vi "DevRef Data Base fg.vi"(6 "DevRef to Get":T11, 9 "Menu":T12) -> (0 "error out":errorcluster, 1 "Selected Sensor":T5, 2 "Selected Encoder":T1={"DevStatus"={"status"=FALSE, "code"=0, "source"=""}, "EncoderIndex"=enum."Invalid", "CounterIndex"=enum."Invalid", "DistancePerCount"=1.0, "Decoding Type"=enum."4x"}, 3 "Selected Solenoid":T8={"DevStatus"={"status"=FALSE, "code"=0, "source"=""}, "Solenoid Module"=enum."Solenoid Module 1", "Forward Solenoid Channel"=enum."Invalid", "Reverse Solenoid Channel"=enum."Invalid"}, 4 "right drive encoder":T1={"DevStatus"={"status"=FALSE, "code"=0, "source"=""}, "EncoderIndex"=enum."Invalid", "CounterIndex"=enum."Invalid", "DistancePerCount"=1.0, "Decoding Type"=enum."4x"}, 5 "left drive encoder":T1={"DevStatus"={"status"=FALSE, "code"=0, "source"=""}, "EncoderIndex"=enum."Invalid", "CounterIndex"=enum."Invalid", "DistancePerCount"=1.0, "Decoding Type"=enum."4x"})   [LabVIEW 2013]
uses:
  typedefs/fg_typedef.ctl
  typedefs/DevRef Type.ctl
  <vilib>/Rock Robotics/WPI/Solenoid/WPI_SolenoidDevRef.ctl
  <vilib>/Rock Robotics/SystemInterfaces/Typedef/FPGA_TypedefSolenoidModule.ctl
  <vilib>/Rock Robotics/WPI/Solenoid/WPI_SolenoidChannel.ctl
  <vilib>/Rock Robotics/WPI/DigitalInput/WPI_DigitalInputDevRef.ctl
  <vilib>/Rock Robotics/SystemInterfaces/DIO/FPGA_DIOChannel.ctl
  <vilib>/Rock Robotics/SystemInterfaces/Typedef/FPGA_TypedefDigitalModule.ctl
  <vilib>/Rock Robotics/WPI/Encoder/WPI_EncoderDevRef.ctl
  <vilib>/Rock Robotics/SystemInterfaces/Encoder/FPGA_EncoderIdx.ctl
  <vilib>/Rock Robotics/SystemInterfaces/Counter/FPGA_CounterCtrSystemIndex.ctl
  <vilib>/Rock Robotics/WPI/Encoder/WPI_EncoderType.ctl
panel:
  # "A Functional Global that stores refnums for \ncommonly used devices \nso as to not need to get them repeatedly"
  # "it is only set once"
  # "Option to Select Also..."
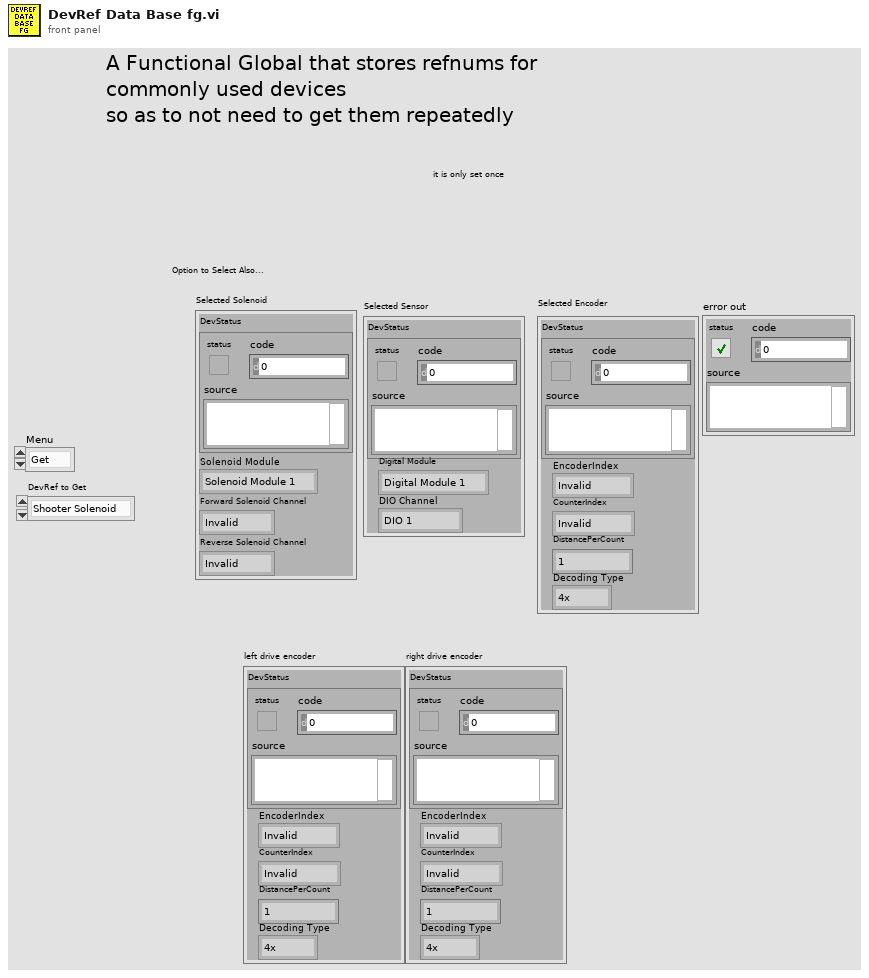
[diagram p1: front panel]
types:
  T1 = typedef "WPI_EncoderDevRef.ctl" = cluster{"DevStatus":errorcluster, "EncoderIndex":T2, "CounterIndex":T3, "DistancePerCount":dbl, "Decoding Type":T4}
  T2 = typedef "FPGA_EncoderIdx.ctl" = enum8{"Enc 0", "Enc 1", "Enc 2", "Enc 3", "Invalid"}
  T3 = typedef "FPGA_CounterCtrSystemIndex.ctl" = enum8{"Ctr 0", "Ctr 1", "Ctr 2", "Ctr 3", "Ctr 4", "Ctr 5", "Ctr 6", "Ctr 7", "Invalid"}
  T4 = typedef "WPI_EncoderType.ctl" = enum16{"1x", "2x", "4x"}
  T5 = typedef "WPI_DigitalInputDevRef.ctl" = cluster{"DevStatus":errorcluster, "DIO Channel":T6, "Digital Module":T7}
  T6 = typedef "FPGA_DIOChannel.ctl" = enum8{"DIO 1", "DIO 2", "DIO 3", "DIO 4", "DIO 5", "DIO 6", "DIO 7", "DIO 8", "DIO 9", "DIO 10", "DIO 11", "DIO 12", "DIO 13", "DIO 14", "Invalid"}
  T7 = typedef "FPGA_TypedefDigitalModule.ctl" = enum16{"Digital Module 1", "Digital Module 2"}
  T8 = typedef "WPI_SolenoidDevRef.ctl" = cluster{"DevStatus":errorcluster, "Solenoid Module":T9, "Forward Solenoid Channel":T10, "Reverse Solenoid Channel":T10}
  T9 = typedef "FPGA_TypedefSolenoidModule.ctl" = enum16{"Solenoid Module 1", "Solenoid Module 2"}
  T10 = typedef "WPI_SolenoidChannel.ctl" = enum8{"Solenoid 1", "Solenoid 2", "Solenoid 3", "Solenoid 4", "Solenoid 5", "Solenoid 6", "Solenoid 7", "Solenoid 8", "Invalid"}
  T11 = typedef "DevRef Type.ctl" = enum16{"Shooter Solenoid", "Latch Solenoid", "Right Up Sensor", "Right Down Sensor", "Hold Sensor", "2 Ball Switch", "Arm Encoder"}
  T12 = typedef "fg_typedef.ctl" = enum16{"Get", "Set"}
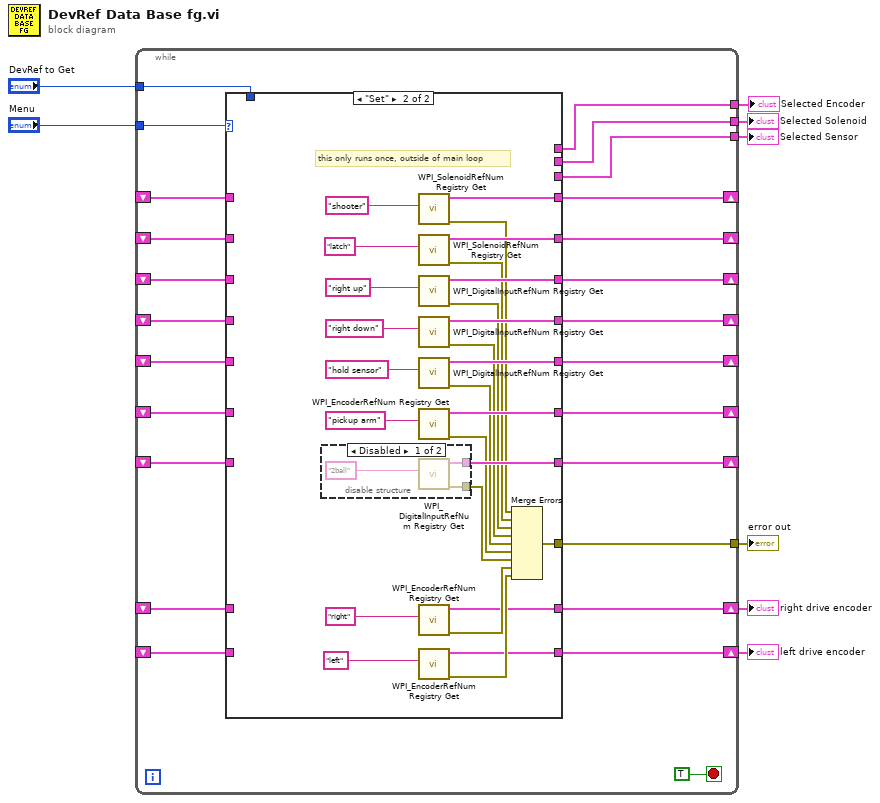
[diagram p0: block diagram]
diagram:
  n1 = while {
    shift-right: [w27] -> _
    shift-left: _ -> [w32]
    shift-right: [w26] -> _
    shift-left: _ -> [w31]
    shift-right: [w25] -> _
    shift-left: _ -> [w29]
    shift-right: [w24] -> _
    shift-left: _ -> [w28]
    tunnel: "Menu" -> [w30]
    shift-right: [w22] -> _
    shift-left: _ -> [w23]
    tunnel: "DevRef to Get" -> [w21]
    tunnel: [w20] -> w6
    tunnel: [w19] -> w5
    shift-right: [w17] -> _
    shift-left: _ -> [w18]
    tunnel: [w16] -> w4
    shift-right: [w15] -> _
    shift-left: _ -> [w14]
    shift-right: [w13] -> w2
    shift-left: _ -> [w10]
    shift-right: [w12] -> w1
    shift-left: _ -> [w9]
    tunnel: [w11] -> w3
    stop <- TRUE stop-if-true
    n2 = case shown="\"Set\"" w30 {
      tunnel: w32 -> [w52 _]
      tunnel: w31 -> [w51 _]
      tunnel: w29 -> [w50 _]
      tunnel: w28 -> [w49 _]
      tunnel: [w41 w124] -> w27
      tunnel: [w42 w123] -> w26
      tunnel: [w43 w122] -> w25
      tunnel: [w44 w121] -> w24
      tunnel: w23 -> [w48 _]
      tunnel: [w45 w120] -> w22
      tunnel: w21 -> [w53 _]
      tunnel: [w47 _] -> w20
      tunnel: [w46 _] -> w19
      tunnel: w18 -> [w40 _]
      tunnel: [w39 w118] -> w17
      tunnel: [w38 _] -> w16
      tunnel: [w37 w117] -> w15
      tunnel: w14 -> [w36 _]
      tunnel: [w35 w105] -> w13
      tunnel: [w34 w104] -> w12
      tunnel: [_ w103] -> w11
      tunnel: w10 -> [w35 _]
      tunnel: w9 -> [w34 _]
      frame "Get", Default {
        # "always get the drive encoders"
        n3 = case shown="\"Shooter Solenoid\", Default" w53 {
          tunnel: w52 -> [w56 w67 w74 w81 w88 w90 w102]
          tunnel: w51 -> [w57 w66 w73 w80 w87 w91 w101]
          tunnel: w50 -> [w58 w65 w72 w79 w86 w92 w100]
          tunnel: w49 -> [w59 w64 w71 w78 w85 w93 w99]
          tunnel: w48 -> [w60 w63 w70 w77 w84 w94 w98]
          tunnel: [w56 w66 _ _ _ _ _] -> w47
          tunnel: [_ _ w72 w78 w84 w89 _] -> w46
          tunnel: [w60 w63 w70 w77 w84 w94 w98] -> w45
          tunnel: [w59 w64 w71 w78 w85 w93 w99] -> w44
          tunnel: [w58 w65 w72 w79 w86 w92 w100] -> w43
          tunnel: [w57 w66 w73 w80 w87 w91 w101] -> w42
          tunnel: [w56 w67 w74 w81 w88 w90 w102] -> w41
          tunnel: w40 -> [w55 w62 w69 w76 w83 w95 w97]
          tunnel: [w55 w62 w69 w76 w83 w95 w97] -> w39
          tunnel: [_ _ _ _ _ _ w97] -> w38
          tunnel: [w54 w61 w68 w75 w82 w89 w96] -> w37
          tunnel: w36 -> [w54 w61 w68 w75 w82 w89 w96]
          frame "Shooter Solenoid", Default {
          }
          frame "Latch Solenoid" {
          }
          frame "Right Up Sensor" {
          }
          frame "Right Down Sensor" {
          }
          frame "Hold Sensor" {
          }
          frame "2 Ball Switch" {
          }
          frame "Arm Encoder" {
          }
        }
      }
      frame "Set" {
        # "this only runs once, outside of main loop"
        n4 = disable-structure shown="Disabled" {
          disable-tunnel: [w132 _] -> w110
          disable-tunnel: [w130 _] -> w117
          frame Disabled {
            n5 = call <vilib>:"WPI_DigitalInputRefNum Registry Get.vi"("refnum name"="2ball") -> ("error out"=w132:errorcluster, "DigitalInputDevRef"=w130:T5)  [unwired: 9 in]
          }
          frame Enabled {
          }
        }
        n6 = call <vilib>:"WPI_SolenoidRefNum Registry Get.vi"("refnum name"="shooter") -> ("error out"=w116:errorcluster, "SolenoidDevRef"=w124:T8)  [unwired: 9 in]
        n7 = call <vilib>:"WPI_SolenoidRefNum Registry Get.vi"("refnum name"="latch") -> ("error out"=w115:errorcluster, "SolenoidDevRef"=w123:T8)  [unwired: 9 in]
        n8 = call <vilib>:"WPI_DigitalInputRefNum Registry Get.vi"("refnum name"="right up") -> ("error out"=w114:errorcluster, "DigitalInputDevRef"=w122:T5)  [unwired: 9 in]
        n9 = call <vilib>:"WPI_DigitalInputRefNum Registry Get.vi"("refnum name"="right down") -> ("error out"=w113:errorcluster, "DigitalInputDevRef"=w121:T5)  [unwired: 9 in]
        n10 = call <vilib>:"WPI_DigitalInputRefNum Registry Get.vi"("refnum name"="hold sensor") -> ("error out"=w112:errorcluster, "DigitalInputDevRef"=w120:T5)  [unwired: 9 in]
        n11 = call <vilib>:"WPI_EncoderRefNum Registry Get.vi"("refnum name"="pickup arm") -> ("error out"=w111:errorcluster, "EncoderDevRef"=w118:T1)  [unwired: 9 in]
        n12 = call <vilib>:"WPI_EncoderRefNum Registry Get.vi"("refnum name"="right") -> ("error out"=w107:errorcluster, "EncoderDevRef"=w105:T1)  [unwired: 9 in]
        n13 = call <vilib>:"WPI_EncoderRefNum Registry Get.vi"("refnum name"="left") -> ("error out"=w106:errorcluster, "EncoderDevRef"=w104:T1)  [unwired: 9 in]
        n14 = Merge Errors(w116, w115, w114, w113, w112, w111, w110, w107, w106) -> (w103:errorcluster)
      }
    }
  }
  "Selected Solenoid" <- w6
  "Selected Sensor" <- w5
  "Selected Encoder" <- w4
  "error out" <- w3
  "right drive encoder" <- w2
  "left drive encoder" <- w1
